vi "GEvt-Generate Complete Log.vi"(0 "CSM Global Log Event":refnum<user-event>, 6 "event data":T1={"Name(\"\" to use uuid)"="", "Current State"="", "Arguments"="", "Source Message"={"‘State"="", "’Arguments"="", "’Error"={"status"=FALSE, "code"=0, "source"=""}}, "Source Module"="", "Complete(T)/Start(F)"=FALSE, "LogType"=enum."State Change"}, 7 "Enable?":bool, 10 "CSM:LogFilter.lvclass":refnum<class "LogFilter.lvclass">) -> (14 "CSM Global Log Event out":refnum<user-event>)   [LabVIEW 2020, in "Communicable State Machine.lvlib"]
uses:
  Communicable State Machine.lvlib
  _CSM_GlobalLog_MSG.ctl
  _CSM_Response Source Message.ctl
  _CSM_GlobalLog_MSG_TYPE.ctl
  LogFilter.lvclass
  Filter Check.vi
  Group Check - CSM.vi
  Group Check - LogType.vi
  Group Check - State.vi
  CSM Check - LogType.vi
  CSM Check - State.vi
  CSM Check - StateType.vi
  Group Check - StateType.vi
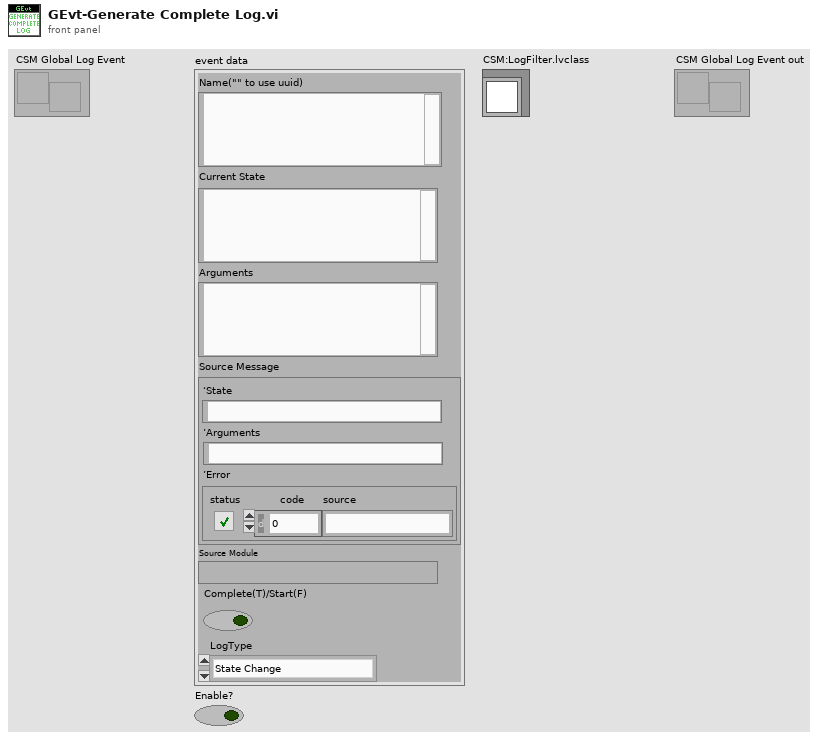
[diagram p1: front panel]
types:
  T1 = typedef "Communicable State Machine.lvlib/_CSM_GlobalLog_MSG.ctl" = cluster{"Name(\"\" to use uuid)":string, "Current State":string, "Arguments":string, "Source Message":T2, "Source Module":string, "Complete(T)/Start(F)":bool, "LogType":T3}
  T2 = typedef "Communicable State Machine.lvlib/_CSM_Response Source Message.ctl" = cluster{"‘State":string, "’Arguments":string, "’Error":errorcluster}
  T3 = typedef "Communicable State Machine.lvlib/_CSM_GlobalLog_MSG_TYPE.ctl" = enum16{"User Log", "State Change", "Status", "Interrupt", "Register", "Unregister", "Error Log", "Module Created", "Module Destroyed"}
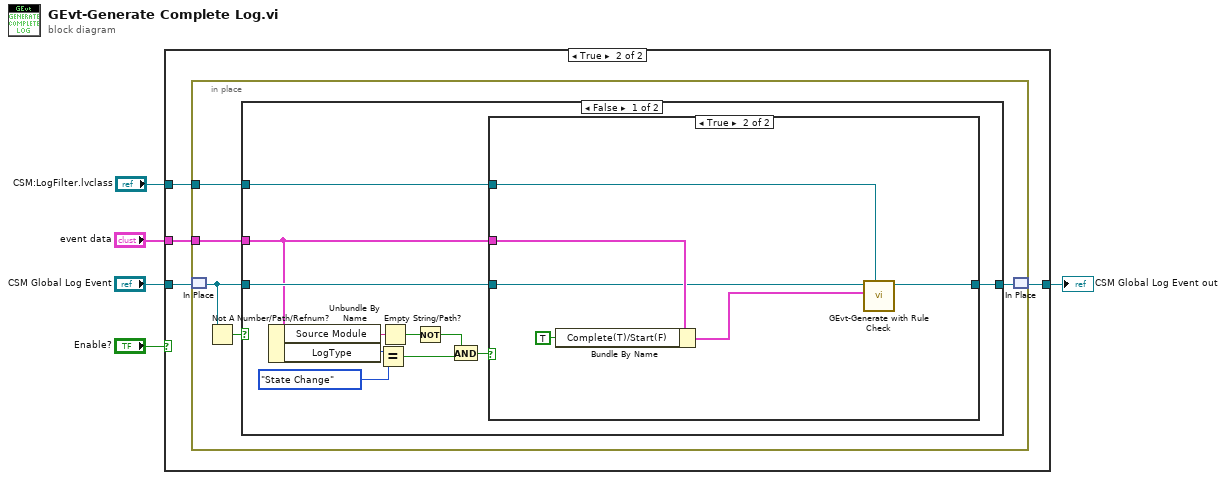
[diagram p0: block diagram]
diagram:
  n1 = case shown="True" "Enable?" {
    tunnel: "CSM Global Log Event" -> [w6 w10]
    tunnel: [w6 w9] -> w4
    tunnel: "event data" -> [_ w8]
    tunnel: "CSM:LogFilter.lvclass" -> [_ w7]
    frame False {
    }
    frame True {
      n2 = in-place {
        in-place-border: w8 -> [w12]
        in-place-border: w7 -> [w11]
        n3 = in-place-match #1(w10) -> (w14:refnum<user-event>)
        n4 = Not A Number/Path/Refnum?(number/path/refnum=w14) -> (NaN/Path/Refnum?=w15:bool)
        n5 = case shown="False" w15 {
          tunnel: w14 -> [w26 w34]
          tunnel: [w25 w34] -> w13
          tunnel: w12 -> [w24 _]
          tunnel: w11 -> [w16 _]
          frame False {
            n6 = Unbundle By Name(w24) -> ("Source Module"=w19:string, "LogType"=w23:T3)
            n7 = Equal?(x=w23, y=_CSM_GlobalLog_MSG_TYPE."State Change") -> (x = y?=w20:bool)
            n8 = Empty String/Path?(string/path=w19) -> (empty?=w18:bool)
            n9 = Not(x=w18) -> (.not. x?=w17:bool)
            n10 = And(x=w17, y=w20) -> (x .and. y?=w21:bool)
            n11 = case shown="True" w21 {
              tunnel: w26 -> [w27 w30]
              tunnel: [w27 w32] -> w25
              tunnel: w24 -> [_ w31]
              tunnel: w16 -> [_ w28]
              frame False {
              }
              frame True {
                n12 = Bundle By Name(cluster=w31, "Complete(T)/Start(F)"=TRUE) -> (w29:T1)
                n13 = call "GEvt-Generate with Rule Check.vi"("LogFilter in"=w28, "event data"=w29, "CSM Global Log Event in"=w30) -> ("CSM Global Log Event out"=w32:refnum<user-event>)  [unwired: 8 in]
              }
            }
          }
          frame True {
          }
        }
        n14 = in-place-match #1(w13) -> (w9:refnum<user-event>)
      }
    }
  }
  "CSM Global Log Event out" <- w4
